vi "Set Parameter Controls.vi"(0 "Controls Mode (Set)":T4=enum."Set Controls", 1 "Para 1 Ref":refnum<vi>, 2 "Para 2 Ref":refnum<vi>, 3 "Para 3 Ref":refnum<vi>, 5 "Para 1":i32=-1, 7 "Para 2":i32=-1, 9 "Para 3":i32=-1, 11 "Error In":errorcluster, 12 "StandConfigCluster":T3, 13 "Controller":T2={"Controller Name"=enum."Kuhnke", "CommSeg"=2, "PWM?"=TRUE, "Frequency"=100, "Low Command"=10.0, "High Command"=90.0, "Stop Command"=10.0, "Command Step"=0.1, "Solenoid Stop?"=FALSE, "Controller?"=TRUE, "Name"="Kuhnke", "Indirect Nonzero CMD"=15.0}, 14 "Min/Max Refs":refnum<vi>[](array[refnum])) -> (15 "Error Out":errorcluster)   [LabVIEW 2019]
uses:
  TypeDef/Parameter Controls Mode.ctl
  TypeDef/StandConfigCluster.ctl
  TypeDef/Controller Names.ctl
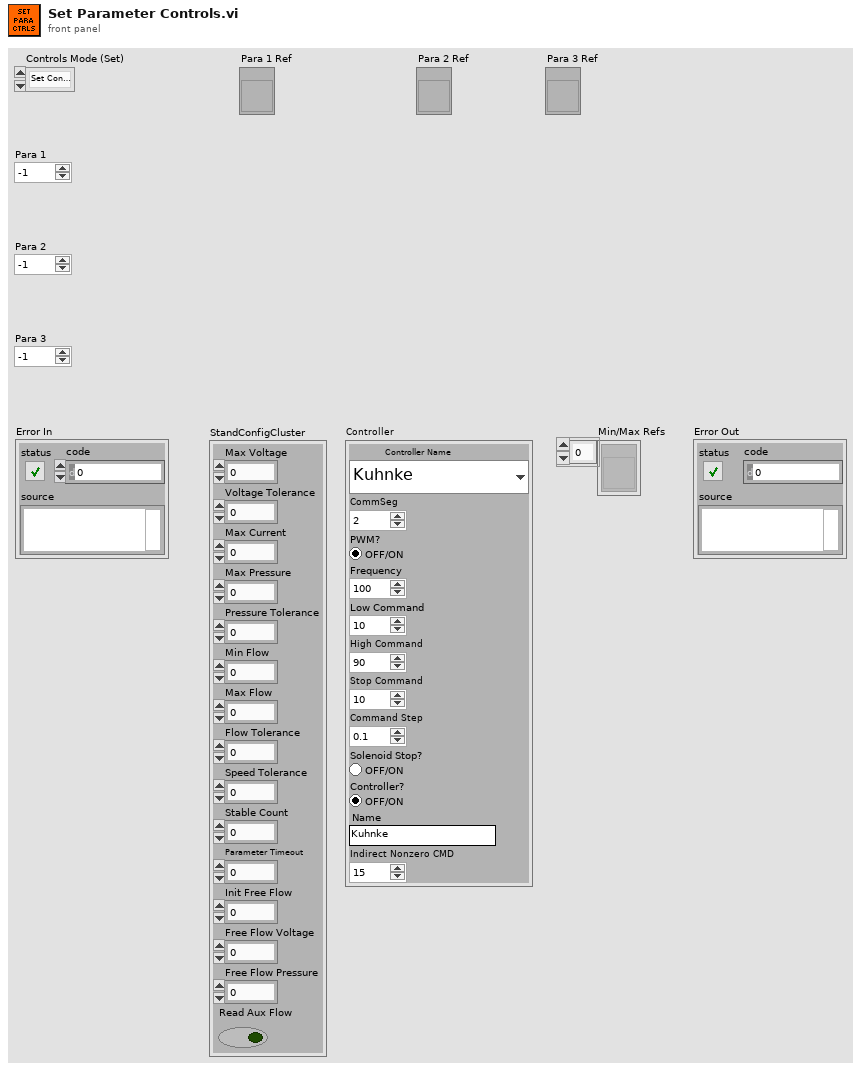
[diagram p1: front panel]
types:
  T1 = typedef "Controller Names.ctl" = enum16{"Kuhnke", "McLaren", "Helbako BLDC", "Conti", "Hella E4LMF", "Hella E4LMD", "Hella E4DCG 20mm", "Hella E4DCG 30mm", "Helbako (old)", "TI PWM", "PSA", "Hella Hyundai Gas", "Hella Hyundai Diesel", "8 Comm", "10 Comm", "8 Comm Hella FCA", "10 Comm Hella FCA", "8 Comm Omron", "10 Comm Omron", "8 Comm Nissan", "10 Comm Nissan", "8 Comm Hella (for FCA)", "Mazda BLDC"}
  T2 = cluster{"Controller Name":T1, "CommSeg":i32, "PWM?":bool, "Frequency":i32, "Low Command":dbl, "High Command":dbl, "Stop Command":dbl, "Command Step":dbl, "Solenoid Stop?":bool, "Controller?":bool, "Name":string, "Indirect Nonzero CMD":dbl}
  T3 = typedef "StandConfigCluster.ctl" = cluster{"Max Voltage":dbl, "Voltage Tolerance":dbl, "Max Current":dbl, "Max Pressure":dbl, "Pressure Tolerance":dbl, "Min Flow":dbl, "Max Flow":dbl, "Flow Tolerance":dbl, "Speed Tolerance":dbl, "Stable Count":dbl, "Parameter Timeout":dbl, "Init Free Flow":dbl, "Free Flow Voltage":dbl, "Free Flow Pressure":dbl, "Read Aux Flow":bool}
  T4 = typedef "Parameter Controls Mode.ctl" = enum16{"Init", "Update Ranges", "Set Controls"}
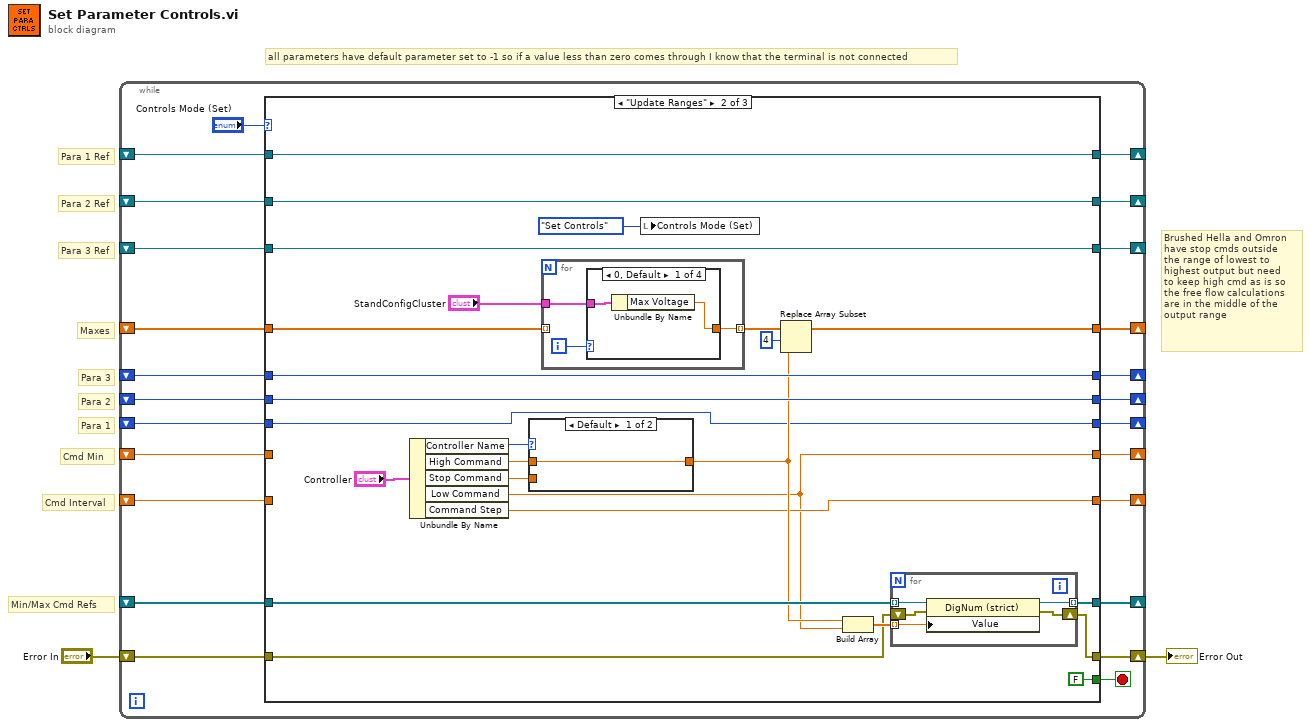
[diagram p0: block diagram]
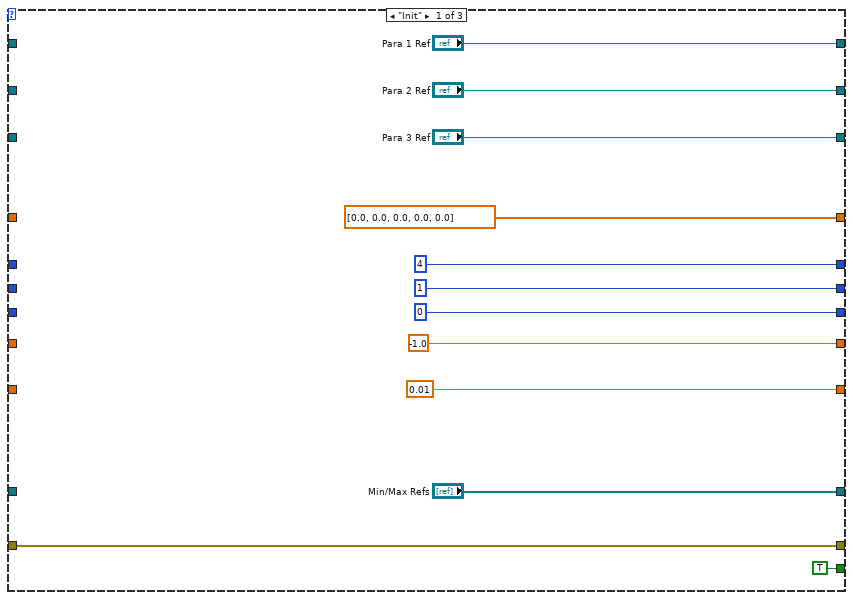
[diagram p2: hidden frame]
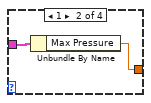
[diagram p3: hidden frame]
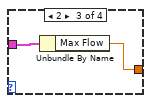
[diagram p4: hidden frame]
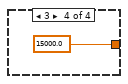
[diagram p5: hidden frame]
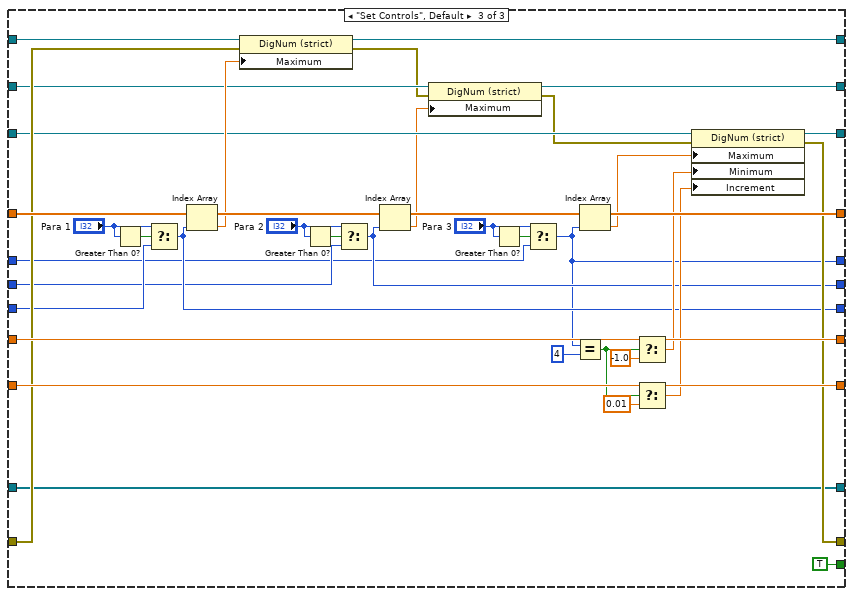
[diagram p7: hidden frame]
diagram:
  # "Min/Max Cmd Refs"
  # "Brushed Hella and Omron\nhave stop cmds outside\nthe range of lowest to \nhighest output but need\nto keep high cmd as is so\nthe free flow calculations\nare in the middle of the\noutput range"
  # "all parameters have default parameter set to -1 so if a value less than zero comes through I know that the terminal is not connected"
  # "Para 3"
  # "Para 2"
  # "Para 1"
  # "Cmd Interval"
  # "Cmd Min"
  # "Maxes"
  # "Para 3 Ref"
  # "Para 2 Ref"
  # "Para 1 Ref"
  n1 = while {
    shift-right: [w25] -> _
    shift-left: _ -> [w22]
    shift-right: [w24] -> _
    shift-left: _ -> [w21]
    shift-right: [w23] -> _
    shift-left: _ -> [w20]
    shift-right: [w18] -> _
    shift-left: _ -> [w19]
    shift-right: [w16] -> _
    shift-left: _ -> [w14]
    shift-right: [w15] -> _
    shift-left: _ -> [w13]
    shift-right: [w11] -> _
    shift-left: _ -> [w12]
    shift-right: [w10] -> _
    shift-left: _ -> [w8]
    shift-right: [w9] -> _
    shift-left: _ -> [w7]
    shift-right: [w5] -> _
    shift-left: _ -> [w4]
    shift-right: [w3] -> w1
    shift-left: "Error In" -> [w17]
    stop <- w6 stop-if-true
    n2 = case shown="\"Update Ranges\"" "Controls Mode (Set)" {
      tunnel: ["Para 1 Ref" w63 w108] -> w25
      tunnel: ["Para 2 Ref" w62 w99] -> w24
      tunnel: ["Para 3 Ref" w61 w98] -> w23
      tunnel: w22 -> [_ w63 w109]
      tunnel: w21 -> [_ w62 w105]
      tunnel: w20 -> [_ w61 w104]
      tunnel: w19 -> [_ w53 w116]
      tunnel: [dbl[] [0.0, 0.0, 0.0, 0.0, 0.0] w41 w116] -> w18
      tunnel: w17 -> [w37 w45 w107]
      tunnel: [w37 w44 w95] -> w3
      tunnel: [-1.0 w42 w113] -> w16
      tunnel: [0.01 w43 w114] -> w15
      tunnel: w14 -> [_ _ w113]
      tunnel: w13 -> [_ _ w114]
      tunnel: w12 -> [_ w60 w82]
      tunnel: [4 w60 w84] -> w11
      tunnel: [1 w59 w87] -> w10
      tunnel: [0 w40 w91] -> w9
      tunnel: w8 -> [_ w59 w83]
      tunnel: w7 -> [_ w40 w90]
      tunnel: [TRUE FALSE TRUE] -> w6
      tunnel: ["Min/Max Refs" w48 w81] -> w5
      tunnel: w4 -> [_ w49 w81]
      frame "Init" {
      }
      frame "Update Ranges" {
        n3 = Unbundle By Name("Controller") -> ("Controller Name"=w56:T1, "High Command"=w55:dbl, "Stop Command"=w54:dbl, "Low Command"=w42:dbl, "Command Step"=w43:dbl)
        n4 = case shown="Default" w56 {
          tunnel: w55 -> [w79 _]
          tunnel: w54 -> [_ w80]
          tunnel: [w79 w80] -> w47
          frame Default {
          }
          frame "10 Comm Hella FCA".."10 Comm Omron" {
          }
        }
        n5 = for {
          tunnel: w53 -> [_] mode=indexing
          tunnel: "StandConfigCluster" -> [w70]
          tunnel: [w69] -> w51 mode=indexing
          i -> [w71]
          n6 = case shown="0, Default" w71 {
            tunnel: w70 -> [w73 w75 w77 _]
            tunnel: [w72 w74 w76 15000.0 ("Max Flow")] -> w69
            frame 0, Default {
              n7 = Unbundle By Name(w73) -> ("Max Voltage"=w72:dbl)
            }
            frame 1 {
              n8 = Unbundle By Name(w75) -> ("Max Pressure"=w74:dbl)
            }
            frame 2 {
              n9 = Unbundle By Name(w77) -> ("Max Flow"=w76:dbl)
            }
            frame 3 {
            }
          }
        }
        n10 = local write "Controls Mode (Set)"(Parameter_Controls_Mode."Set Controls" ("Controls Mode (Set)")) -> ()
        n11 = Replace Array Subset(array=w51, new element=w47, index=4) -> (w41:dbl[])
        n12 = Build Array(w47, w42) -> (w46:dbl[])
        n13 = for {
          tunnel: w49 -> [w68] mode=indexing
          tunnel: [w67] -> w48 mode=indexing
          tunnel: w46 -> [w66] mode=indexing
          shift-right: [w64] -> w44
          shift-left: w45 -> [w65]
          n14 = property class="DigNum (strict)"(reference=w68, error in=w65, "Value"=w66) -> (reference out=w67:refnum<vi>, error out=w64:errorcluster)
        }
      }
      frame "Set Controls", Default {
        n15 = Greater Than 0?(x="Para 1") -> (x > 0?=w93:bool)
        n16 = Select(t="Para 1", s=w93, f=w90) -> (s? t:f=w91:i32)
        n17 = Index Array(array=w116, index=w91) -> (element=w106:dbl)
        n18 = property class="DigNum (strict)"(reference=w109, error in=w107, "Maximum"=w106) -> (reference out=w108:refnum<vi>, error out=w97:errorcluster)
        n19 = Greater Than 0?(x="Para 2") -> (x > 0?=w89:bool)
        n20 = Select(t="Para 2", s=w89, f=w83) -> (s? t:f=w87:i32)
        n21 = Index Array(array=w116, index=w87) -> (element=w103:dbl)
        n22 = property class="DigNum (strict)"(reference=w105, error in=w97, "Maximum"=w103) -> (reference out=w99:refnum<vi>, error out=w96:errorcluster)
        n23 = Greater Than 0?(x="Para 3") -> (x > 0?=w86:bool)
        n24 = Select(t="Para 3", s=w86, f=w82) -> (s? t:f=w84:i32)
        n25 = Equal?(x=w84, y=4) -> (x = y?=w110:bool)
        n26 = Index Array(array=w116, index=w84) -> (element=w102:dbl)
        n27 = Select(t=w113, s=w110, f=-1.0) -> (s? t:f=w101:dbl)
        n28 = Select(t=w114, s=w110, f=0.01) -> (s? t:f=w100:dbl)
        n29 = property class="DigNum (strict)"(reference=w104, error in=w96, "Maximum"=w102, "Minimum"=w101, "Increment"=w100) -> (reference out=w98:refnum<vi>, error out=w95:errorcluster)
      }
    }
  }
  "Error Out" <- w1
